vi "Increment.vi"(8 "error in (no error)":errorcluster, 10 "Numeric":dbl, 11 "TestActor in":refnum<class "TestActor.lvclass">) -> (0 "error out":errorcluster, 3 "TestActor out":refnum<class "TestActor.lvclass">)   [LabVIEW 2011, in "TestActor.lvclass"]
uses:
  TestActor.lvclass
  TestActor.lvclass/TestActor.ctl
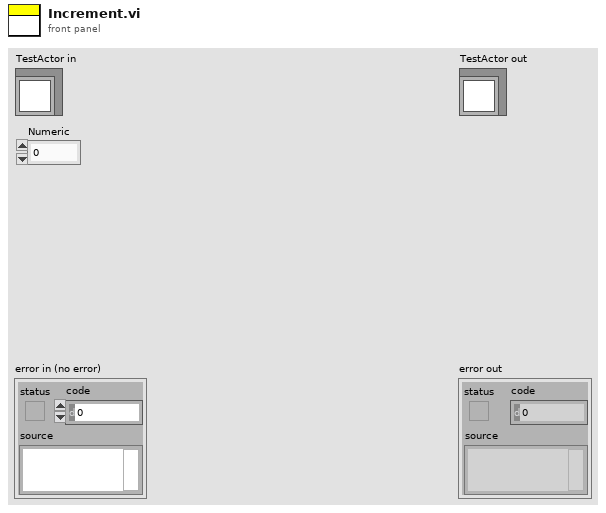
[diagram p1: front panel]
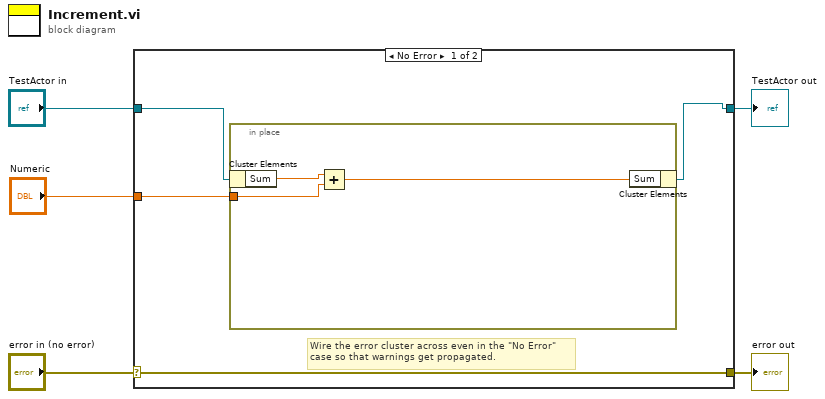
[diagram p0: block diagram]
diagram:
  n1 = case shown="No Error" "error in (no error)" {
    selector: "error in (no error)" -> [w9 w14]
    tunnel: [w9 w14] -> w4
    tunnel: [w7 w13] -> w2
    tunnel: "TestActor in" -> [w8 w13]
    tunnel: "Numeric" -> [w6 _]
    frame No Error {
      # "Wire the error cluster across even in the \"No Error\"\ncase so that warnings get propagated."
      n2 = in-place {
        in-place-border: w6 -> [w11]
        n3 = in-place-cluster #1(w8) -> ("Sum"=w12:dbl)
        n4 = Add(x=w12, y=w11) -> (x+y=w10:dbl)
        n5 = in-place-cluster #1("Sum"=w10) -> (w7:refnum<class "TestActor.lvclass">)
      }
    }
    frame Error {
    }
  }
  "error out" <- w4
  "TestActor out" <- w2
